vi "sendSimpleEmail.vi"(8 "error in (no error)":errorcluster, 11 "args":T1) -> (0 "error out":errorcluster, 3 "sendSimpleEmail_lv_response":T2)   [LabVIEW 2020]
uses:
  mailersend_typedefs/sendSimpleEmail_lv_response.ctl
  mailersend_typedefs/sendSimpleEmail_args.ctl
panel:
  out "value":cluster{"info":string, "status":bool}
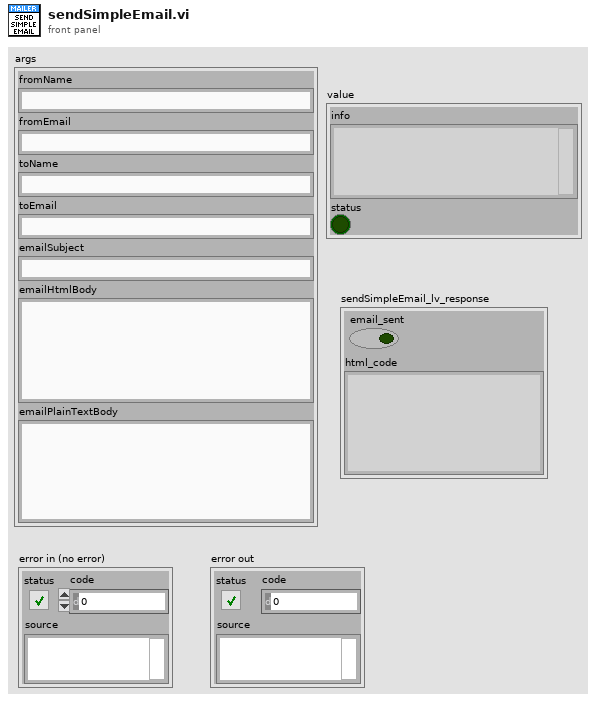
[diagram p1: front panel]
types:
  T1 = typedef "sendSimpleEmail_args.ctl" = cluster{"fromName":string, "fromEmail":string, "toName":string, "toEmail":string, "emailSubject":string, "emailHtmlBody":string, "emailPlainTextBody":string}
  T2 = typedef "sendSimpleEmail_lv_response.ctl" = cluster{"email_sent":bool, "html_code":string}
  T3 = cluster{"func":string, "return_expected":bool, "args":T1}
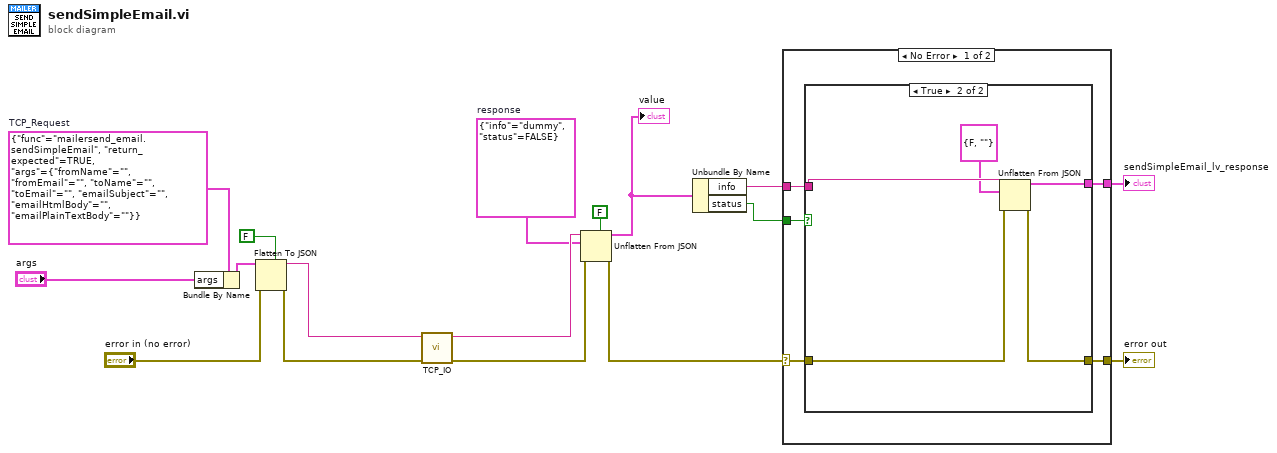
[diagram p0: block diagram]
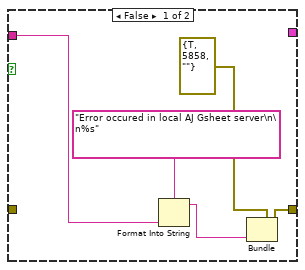
[diagram p2: hidden frame]
diagram:
  w10 = cluster{"info":string, "status":bool} {"info"="dummy", "status"=FALSE}  # response
  w9 = T3 {"func"="mailersend_email.sendSimpleEmail", "return_expected"=TRUE, "args"={"fromName"="", "fromEmail"="", "toName"="", "toEmail"="", "emailSubject"="", "emailHtmlBody"="", "emailPlainTextBody"=""}}  # TCP_Request
  n1 = Bundle By Name(cluster=w9, "args"="args") -> (w2:T3)
  n2 = Flatten To JSON(enable LabVIEW extensions? (T)=FALSE, anything=w2, error in (no error)="error in (no error)") -> (JSON string=w16:string, 11:w11:errorcluster)
  n3 = call "TCP_IO.vi"("error in (no error)"=w11, "Request to Server (JSON)"=w16) -> ("error out"=w13:errorcluster, "Response from Server (JSON)"=w17:string)  [unwired: 8 in]
  n4 = Unflatten From JSON(enable LabVIEW extensions? (T)=FALSE, JSON string=w17, type and defaults=w10, error in (no error)=w13) -> (value=w8:cluster{"info":string, "status":bool}, error out=w6:errorcluster)  [unwired: 3 in]
  "value" <- w8
  n5 = Unbundle By Name(w8) -> ("info"=w7:string, "status"=w5:bool)
  n6 = case shown="No Error" w6 {
    selector: w6 -> [w21 w33]
    tunnel: w7 -> [w22 _]
    tunnel: w5 -> [w20 _]
    tunnel: [w19 _] -> w3
    tunnel: [w18 w33] -> w4
    frame No Error {
      n7 = case shown="True" w20 {
        tunnel: w22 -> [w26 w32]
        tunnel: w21 -> [_ w30]
        tunnel: [_ w29] -> w19
        tunnel: [w24 w28] -> w18
        frame False {
          n8 = Format Into String(format string="Error occured in local AJ Gsheet server\n\n%s", w26) -> (resulting string=w23:string)  [unwired: 2 in, 1 out]
          n9 = Bundle(cluster=errorcluster {"status"=TRUE, "code"=5858, "source"=""} ("error IO"), "source"=w23) -> (w24:errorcluster)  [unwired: 2 in]
        }
        frame True {
          n10 = Unflatten From JSON(JSON string=w32, type and defaults=T2 {"email_sent"=FALSE, "html_code"=""}, error in (no error)=w30) -> (value=w29:T2, error out=w28:errorcluster)  [unwired: 4 in]
        }
      }
    }
    frame Error {
    }
  }
  "error out" <- w4
  "sendSimpleEmail_lv_response" <- w3
